vi "Display Table Mode.vi"(8 "error in (no error)":errorcluster, 9 "Top Line Number (1)":i32=1 min=1 max=401, 10 "Unit Display (T:On)":bool=TRUE, 11 "VISA resource name":refnum<visa-resource-name>) -> (0 "error out":errorcluster, 3 "VISA resource name out":refnum<visa-resource-name>)   [LabVIEW 2010, in "Agilent 4194.lvlib"]
doc: "This function sets the display parameters effective for table mode.\n\nNotes:\n\n(1) This function is valid for Table mode setting only."
uses:
  <instrlib>/Agilent 4194/Agilent 4194.lvlib
panel:
  # "On"
  # "Off"
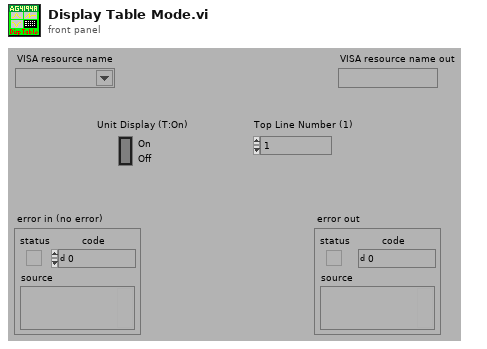
[diagram p1: front panel]
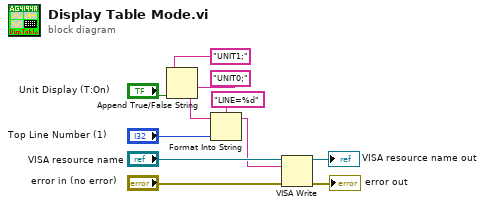
[diagram p0: block diagram]
diagram:
  n1 = Append True/False String(1:"Unit Display (T:On)", 2:"UNIT0;" ("false string"), 3:"UNIT1;" ("false string")) -> (0:w2:string)  [unwired: 1 in]
  n2 = Format Into String(format string="LINE=%d" ("false string"), initial string=w2, "Top Line Number (1)") -> (resulting string=w1:string)  [unwired: 1 in, 1 out]
  n3 = VISA Write(VISA resource name="VISA resource name", write buffer=w1, error in (no error)="error in (no error)") -> (VISA resource name out=→"VISA resource name out":refnum<visa-resource-name>, error out=→"error out":errorcluster)  [unwired: 1 out]
